vi "MyVI.vi"   [LabVIEW 2018, in "MyClass.lvclass"]
uses:
  MyClass.lvclass
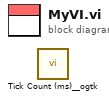
[diagram p0: block diagram]
diagram:
  n1 = call <userlib>:"Tick Count (ms)__ogtk.vi"() -> ()  [unwired: 10 in, 2 out]
